vi "Get OpMode.vi"(4 "error in (no error)":errorcluster) -> (0 "error out":errorcluster, 3 "SimMode":bool)   [LabVIEW 2023]
uses:
  <vilib>/Utility/config.llb/Read Key (I32).vi
  <vilib>/Utility/config.llb/NI_LVConfig.lvlib
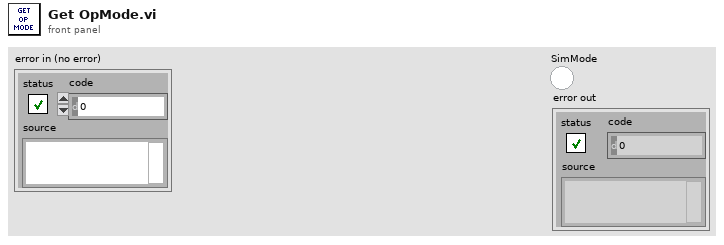
[diagram p1: front panel]
types:
  T1 = typedef "NI_LVConfig.lvlib/Config Data RefNum.ctl" = refnum<k1>
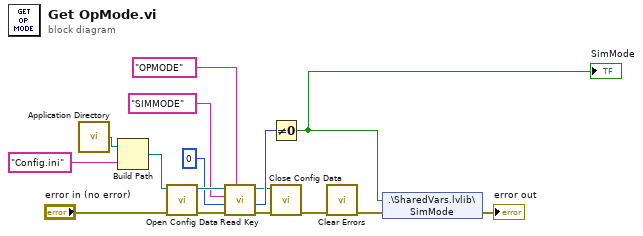
[diagram p0: block diagram]
diagram:
  n1 = call <vilib>:"Application Directory.vi"() -> ("Application Directory"=w16:path)
  n2 = Build Path(base path=w16, name or relative path="Config.ini") -> (appended path=w14:path)
  n3 = call <vilib>:"Open Config Data.vi"("error in (no error)"="error in (no error)", "configuration file path"=w14) -> ("error out"=w11:errorcluster, "refnum"=w12:T1)  [unwired: 7 in, 1 out]
  n4 = call-poly <vilib>:"Read Key.vi"("section"="OPMODE", "error in (no error)"=w11, "default value"=0, "key"="SIMMODE", "refnum"=w12) -> ("error out"=w5:errorcluster, "value"=w7:i32, "refnum out"=w6:T1)  [unwired: 3 in, 1 out]
  n5 = Not Equal To 0?(x=w7) -> (x != 0?=w1:bool)
  "SimMode" <- w1
  n6 = call <vilib>:"Close Config Data.vi"("error in (no error)"=w5, "refnum"=w6) -> ("error out"=w4:errorcluster)  [unwired: 8 in, 1 out]
  n7 = call <vilib>:"Clear Errors.vi"("error in (no error)"=w4) -> ("error out"=w3:errorcluster)  [unwired: 5 in, 1 out]
  n8 = shared-variable ".\\SharedVars.lvlib\\SimMode"(w1, error in=w3) -> (error out=→"error out":errorcluster)
